vi "Write Tab Control.vi"(8 "error in":errorcluster, 10 "Value":string[](array[string]), 11 "Tab Control in":refnum<vi>) -> (0 "error out":errorcluster, 3 "Tab Control out":refnum<vi>)   [LabVIEW 2020, in "G-Unicode.lvlib"]
uses:
  G-Unicode.lvlib
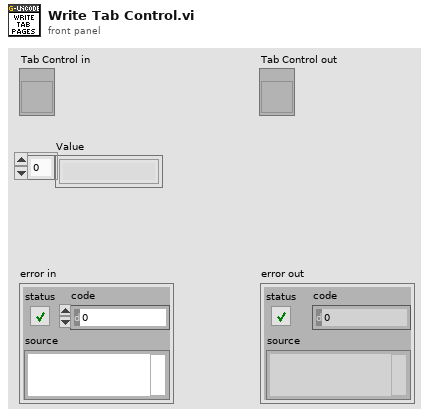
[diagram p1: front panel]
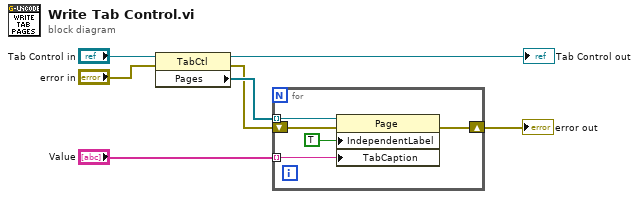
[diagram p0: block diagram]
diagram:
  n1 = property class="TabCtl"(reference="Tab Control in", error in="error in") -> (reference out=→"Tab Control out":refnum<vi>, error out=w3:errorcluster, "Pages"=w7:refnum<vi>[])
  n2 = for {
    tunnel: w7 -> [w12] mode=indexing
    shift-right: [w10] -> w1
    shift-left: w3 -> [w11]
    tunnel: "Value" -> [w8] mode=indexing
    n3 = property class="Page"(reference=w12, error in=w11, "IndependentLabel"=TRUE ("Independent Label"), "TabCaption"=w8) -> (error out=w10:errorcluster)  [unwired: 1 out]
  }
  "error out" <- w1
